vi "ReadButtonBar.vi"(8 "Error In":errorcluster, 11 "reference in":refnum<class "TemplateGUI.lvclass">) -> (0 "Error Out":errorcluster, 2 "ButtonBar":refnum<class "ButtonCollection.lvclass"> caption="Object Out", 3 "reference out":refnum<class "TemplateGUI.lvclass">)   [LabVIEW 2021]
uses:
  TemplateGUI.lvclass/TemplateGUI.ctl
  TemplateGUI.lvclass
  VerticalButtonBar/ButtonCollection/ButtonCollection.lvclass
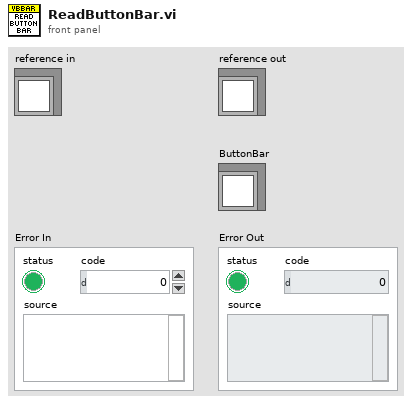
[diagram p1: front panel]
types:
  T1 = typedef "TemplateGUI.lvclass/ObjectAttributes.ctl" = cluster{"Interfaces":cluster{"Dummys":refnum<class>}, "Locals":cluster{"Dummy":bool}, "Persistent":cluster{"Dummy":bool}}
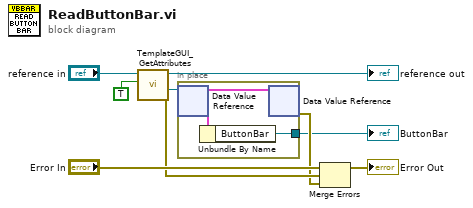
[diagram p0: block diagram]
diagram:
  n1 = call "TemplateGUI_GetAttributes.vi"("OnlyGetDvrReference(False)"=TRUE, "reference in"="reference in") -> ("error out"=w6:errorcluster, "DataRef"=w3:refnum<data-value>, "reference out"=→"reference out":refnum<class "TemplateGUI.lvclass">)  [unwired: 6 in, 1 out]
  n2 = in-place {
    in-place-border: [w11] -> w1
    n3 = in-place-dvr #1(w3) -> (w10:T1)  [unwired: 1 out]
    n4 = Unbundle By Name(w10) -> ("ButtonBar"=w11:refnum<class "ButtonCollection.lvclass">)
    n5 = in-place-dvr #1(w10) -> (w2:errorcluster)  [unwired: 1 out]
  }
  "ButtonBar" <- w1
  n6 = Merge Errors("Error In", w6, w2) -> (→"Error Out":errorcluster)
